vi "Prompt for Step--UI Interlocks.vi"(8 "error in (no error)":errorcluster, 10 "Control Ref Map":map{string, refnum<vi>}(c390), 11 "Numeric Assertion in":refnum<class "Numeric Assertion.lvclass">) -> (0 "error out":errorcluster, 2 "Error List":string[](array[string]), 3 "Numeric Assertion out":refnum<class "Numeric Assertion.lvclass">)   [LabVIEW 2020, in "MacroAssert.lvlib" / "Numeric Assertion.lvclass"]
doc: "Enables or disables buttons within the \"Prompt for Step\" VI according to the current state of the system."
uses:
  Numeric Assertion.lvclass
  Numeric Assertion.lvclass/Numeric Assertion.ctl
  MacroAssert.lvlib
  Support/Get Control Reference by Label (1D STR).vi
  Numeric Assertion Type.ctl
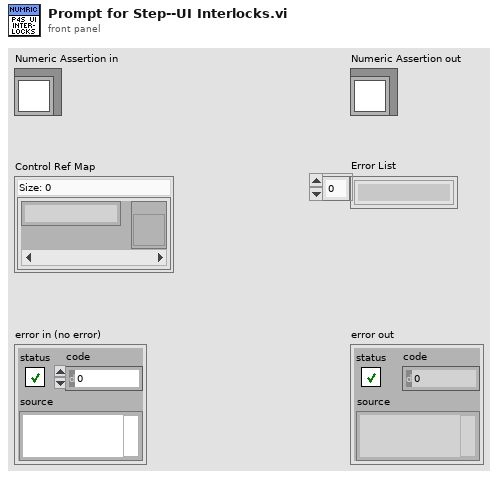
[diagram p1: front panel]
types:
  T1 = typedef "MacroAssert.lvlib/Numeric Assertion.lvclass/Numeric Assertion Type.ctl" = enum16{"Numeric Ctl Value", "Array Ctl Size", "Ctl Width Property", "Ctl Height Property", "VI Width", "VI Height", "Window Width", "Window Height", "Window Scale", "Number of Monitors"}
  T2 = enum8{"Enabled", "Disabled", "Disabled and Grayed Out"}
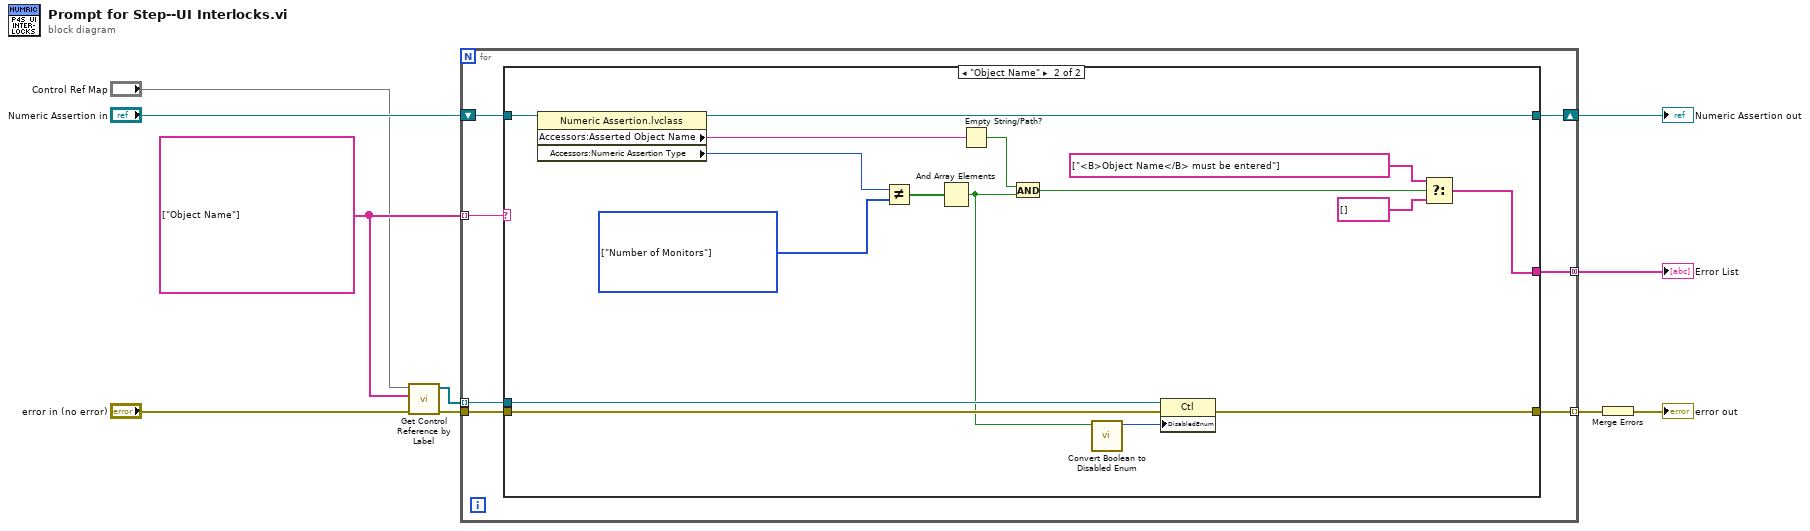
[diagram p0: block diagram]
diagram:
  w9 = string[] ["Object Name"]
  n1 = call-poly "Get Control Reference by Label.vi"("error in (no error)"="error in (no error)", "Control Names"=w9, "Control Ref Map"="Control Ref Map") -> ("error out"=w8:errorcluster, "Control Refs"=w7:refnum<vi>[])  [unwired: 6 in, 1 out]
  n2 = for {
    shift-right: [w14] -> w2
    shift-left: "Numeric Assertion in" -> [w17]
    tunnel: w9 -> [w16] mode=indexing
    tunnel: [w15] -> w10 mode=indexing
    tunnel: w8 -> [w13]
    tunnel: w7 -> [w12] mode=indexing
    tunnel: [w11] -> w1 mode=concatenating
    n3 = case shown="\"Object Name\"" w16 {
      tunnel: w17 -> [w18 w35]
      tunnel: w13 -> [w19 w33]
      tunnel: [w19 w32] -> w15
      tunnel: [w18 w34] -> w14
      tunnel: w12 -> [_ w31]
      tunnel: [_ w25] -> w11
      frame Default {
      }
      frame "Object Name" {
        w30 = T1[] [enum."Number of Monitors"] items=["Numeric Ctl Value", "Array Ctl Size", "Ctl Width Property", "Ctl Height Property", "VI Width", "VI Height", "Window Width", "Window Height", "Window Scale", "Number of Monitors"]
        n4 = property class="Numeric Assertion.lvclass"(reference=w35) -> (reference out=w34:refnum<class "Numeric Assertion.lvclass">, "Accessors:Asserted Object Name"=w22:string, "Accessors:Numeric Assertion Type"=w23:T1)  [unwired: 1 in, 1 out]
        n5 = Not Equal?(x=w23, y=w30) -> (x != y?=w29:bool[])
        n6 = And Array Elements(Boolean array=w29) -> (logical AND=w24:bool)
        n7 = Empty String/Path?(string/path=w22) -> (empty?=w21:bool)
        n8 = And(x=w21, y=w24) -> (x .and. y?=w20:bool)
        n9 = call "Convert Boolean to Disabled Enum.vi"("Enabled?"=w24) -> ("Disabled Enum"=w28:T2)  [unwired: 10 in]
        n10 = property class="Ctl"(reference=w31, error in=w33, "DisabledEnum"=w28) -> (error out=w32:errorcluster)  [unwired: 1 out]
        n11 = Select(t=string[] ["<B>Object Name</B> must be entered"], s=w20, f=string[] []) -> (s? t:f=w25:string[])
      }
    }
  }
  "Numeric Assertion out" <- w2
  "Error List" <- w1
  n12 = Merge Errors(w10) -> (→"error out":errorcluster)
